vi "LastStepMsgTABLEParser.vi"(5 "Color Arr Refnum":refnum<vi>, 6 "Tbl Refnum":refnum<vi>, 7 "Out MSG Names":string[](array[string]), 8 "old msg counter":i32, 9 "Codes":i32[](array[numeric]), 10 "Msg Array":T1(array[cluster])) -> (2 "code":i32[](array[numeric]), 3 "current msg counter":i32)   [LabVIEW 2010]
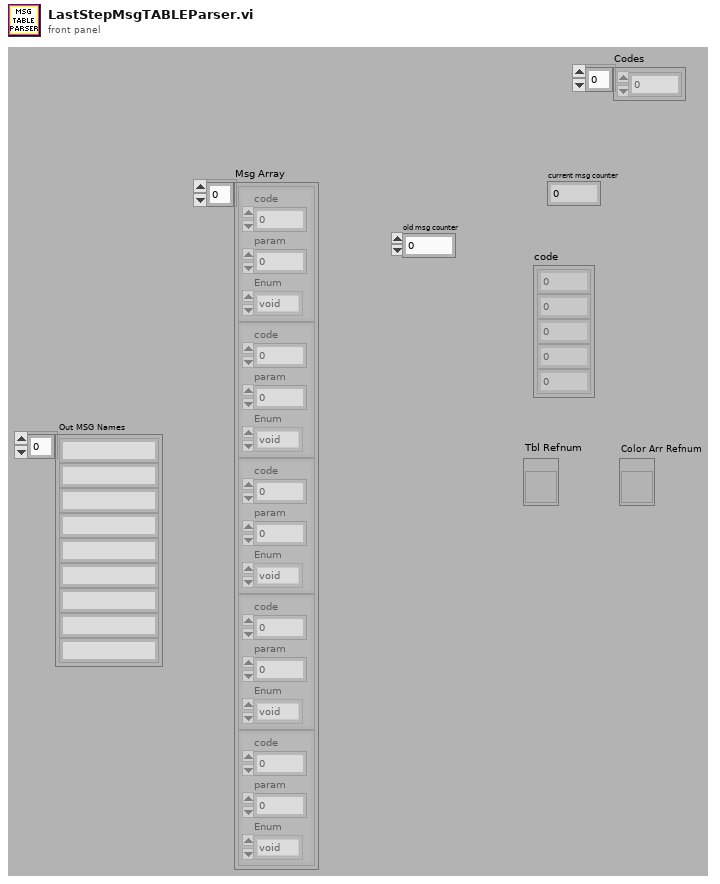
[diagram p1: front panel]
types:
  T1 = cluster{"code":i16, "param":i32, "Enum":enum16{"void", "byte", "int", "float"}}[]
  T2 = cluster{"code":i32, "param":i32, "Enum":enum16{"void", "byte", "int", "float"}}
  T3 = cluster{"code":i16, "param":i32, "Enum":enum16{"void", "byte", "int", "float"}}
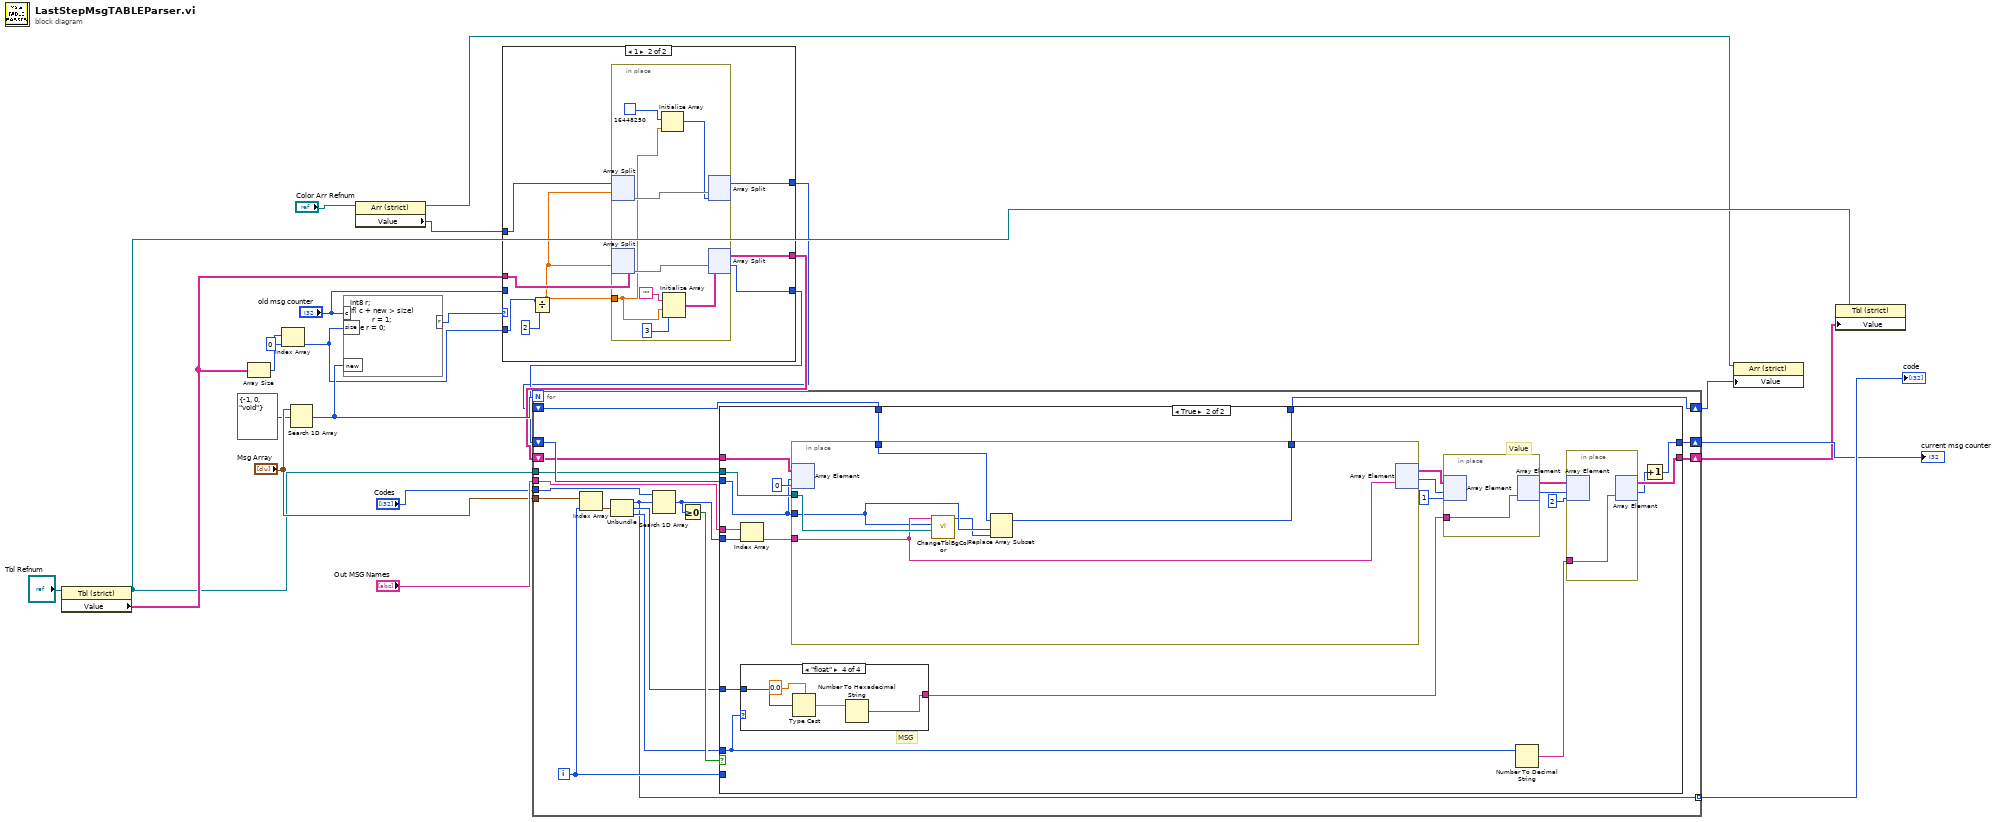
[diagram p0: block diagram]
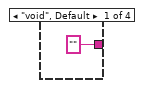
[diagram p4: hidden frame]
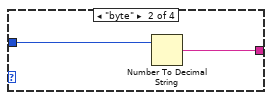
[diagram p5: hidden frame]
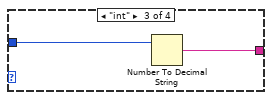
[diagram p6: hidden frame]
diagram:
  n1 = property class="Tbl (strict)"(reference="Tbl Refnum") -> (reference out=w6:refnum<vi>, "Value"=w15:string[][])  [unwired: 1 in, 1 out]
  n2 = Array Size(array=w15) -> (size(s)=w9:i32[])
  n3 = Index Array(array=w9, index=0) -> (element=w7:i32)
  n4 = Search 1D Array(1D array="Msg Array", element=T2 {"code"=-1, "param"=0, "Enum"=enum."void"} ("Cluster")) -> (index of element=w14:i32)  [unwired: 1 in]
  n5 = formula code="int8 r;\nif( c + new > size)\n           r = 1;\nelse r = 0;"("c"="old msg counter", "size"=w7, "new"=w14) -> ("r"=w16:i8)
  n6 = property class="Arr (strict)"(reference="Color Arr Refnum") -> (reference out=w2:refnum<vi>, "Value"=w4:u32[])  [unwired: 1 in, 1 out]
  n7 = case shown="1" w16 {
    tunnel: w15 -> [w26 w32]
    tunnel: w7 -> [_ w34]
    tunnel: [w26 w31] -> w13
    tunnel: "old msg counter" -> [w25 _]
    tunnel: [w25 w30] -> w11
    tunnel: w4 -> [w24 w29]
    tunnel: [w24 w27] -> w3
    frame 0, Default {
    }
    frame 1 {
      n8 = Divide(x=w34, y=2) -> (x/y=w28:dbl)
      n9 = in-place {
        in-place-border: w28 -> [w36]
        n10 = in-place-split #1(w29, w28) -> (w38:u32[])  [unwired: 1 out]
        n11 = in-place-split #2(w32, w28) -> (w42:string[][])  [unwired: 1 out]
        n12 = Initialize Array(u32 16448250 ("Success"), w36) -> (w35:u32[])
        n13 = Initialize Array("", w36, 3 ("dimension size")) -> (w40:string[][])
        n14 = in-place-split #1(w38, w35) -> (w27:u32[])  [unwired: 1 out]
        n15 = in-place-split #2(w42, w40) -> (w31:string[][], w30:i32)
      }
    }
  }
  n16 = for {
    N: w14 -> [_]
    tunnel: "Msg Array" -> [w54]
    tunnel: [w50] -> w22 mode=indexing
    tunnel: "Codes" -> [w57]
    tunnel: "Out MSG Names" -> [w56]
    shift-right: [w48] -> w18
    shift-left: w11 -> [w49]
    shift-right: [w46] -> w10
    shift-left: w13 -> [w47]
    tunnel: w6 -> [w45]
    shift-right: [w43] -> w1
    shift-left: w3 -> [w44]
    i -> [w53]
    n17 = Index Array(array=w54, index=w53) -> (element=w52:T3)
    n18 = Unbundle(w52) -> ("code"=w50:i16, "param"=w55:i32, "Enum"=w51:enum16{"void", "byte", "int", "float"})
    n19 = Search 1D Array(1D array=w57, element=w50) -> (index of element=w58:i32)  [unwired: 1 in]
    n20 = Greater Or Equal To 0?(x=w58) -> (x >= 0?=w59:bool)
    n21 = case shown="True" w59 {
      tunnel: w56 -> [_ w84]
      tunnel: w58 -> [_ w83]
      tunnel: w55 -> [_ w82]
      tunnel: w53 -> [_ _]
      tunnel: w51 -> [_ w70]
      tunnel: w49 -> [w62 w65]
      tunnel: [w62 w81] -> w48
      tunnel: w47 -> [w61 w80]
      tunnel: [w61 w68] -> w46
      tunnel: w45 -> [_ w66]
      tunnel: w44 -> [w60 w64]
      tunnel: [w60 w63] -> w43
      frame False {
      }
      frame True {
        # "Value"
        # "MSG"
        n22 = Index Array(array=w84, index=w83) -> (element=w78:string)
        n23 = case shown="\"float\"" w70 {
          tunnel: w82 -> [_ w95 w97 w101]
          tunnel: ["" ("decimal integer string") w94 w96 w98] -> w74
          frame "void", Default {
          }
          frame "byte" {
            n24 = Number To Decimal String(number=w95) -> (decimal integer string=w94:string)  [unwired: 1 in]
          }
          frame "int" {
            n25 = Number To Decimal String(number=w97) -> (decimal integer string=w96:string)  [unwired: 1 in]
          }
          frame "float" {
            n26 = Type Cast(type=0.0 ("default (0 dbl)"), x=w101) -> (*(type *) &x=w99:dbl)
            n27 = Number To Hexadecimal String(2:w99) -> (0:w98:string)  [unwired: 1 in]
          }
        }
        n28 = in-place {
          in-place-border: w78 -> [w91]
          in-place-border: w66 -> [w92]
          in-place-border: w65 -> [w89]
          in-place-border: w64 -> [w90]
          in-place-border: [w87] -> w63
          n29 = in-place-array #3(w80, w65, 0) -> ()  [unwired: 1 out]
          n30 = call "ChangeTblBgColor.vi"("reference"=w92, "Row"=w89, "input string"=w91) -> ("Color"=w88:u32)  [unwired: 5 in]
          n31 = Replace Array Subset(array=w90, new element=w88, index=w89) -> (w87:u32[])
          n32 = in-place-array #3(w91) -> (w75:string[][], w77:i32)  [unwired: 1 out]
        }
        n33 = in-place {
          in-place-border: w74 -> [w86]
          n34 = in-place-array #4(w75, w77, 1) -> ()  [unwired: 1 out]
          n35 = in-place-array #4(w86) -> (w73:string[][], w72:i32)  [unwired: 1 out]
        }
        n36 = Number To Decimal String(number=w70) -> (decimal integer string=w69:string)  [unwired: 1 in]
        n37 = in-place {
          in-place-border: w69 -> [w85]
          n38 = in-place-array #5(w73, w72, 2) -> ()  [unwired: 1 out]
          n39 = in-place-array #5(w85) -> (w68:string[][], w67:i32)  [unwired: 1 out]
        }
        n40 = Increment(x=w67) -> (x+1=w81:i32)
      }
    }
  }
  "code" <- w22
  "current msg counter" <- w18
  n41 = property class="Arr (strict)"(reference=w2, "Value"=w1) -> ()  [unwired: 1 in, 2 out]
  n42 = property class="Tbl (strict)"(reference=w6, "Value"=w10) -> ()  [unwired: 1 in, 2 out]
